vi "Get Emb URL.vi"(11 "Embedding Model URL in":string) -> (3 "Embedding Model URL out":string)   [LabVIEW 2023, in "LabVIEW RAG.lvlib"]
uses:
  LabVIEW RAG.lvlib
  AI RAG Globals.vi
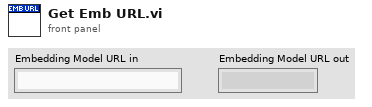
[diagram p1: front panel]
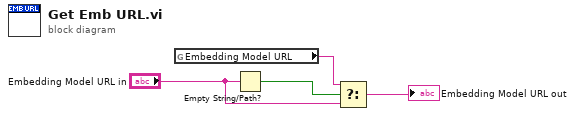
[diagram p0: block diagram]
diagram:
  n1 = global read "AI RAG Globals.vi" "Embedding Model URL"() -> (w4:string)
  n2 = Empty String/Path?(string/path="Embedding Model URL in") -> (empty?=w3:bool)
  n3 = Select(t=w4, s=w3, f="Embedding Model URL in") -> (s? t:f=→"Embedding Model URL out":string)
